vi "TestExec.Config, Dialog, Setup Station Config.vi"(7 "Error if EXE does not exist":bool, 8 "Error if File Doesn't Exist":bool, 9 "Create File if Doesn't Exist":bool, 11 "Path":path=path "C:/MTE/Test Executive/Config") -> (0 "error out":errorcluster, 1 "Station IP Port":i32, 2 "Station Name":string, 3 "Sta Exe Path":path)   [LabVIEW 2018]
uses:
  <vilib>/Utility/config.llb/Read Key (String).vi
  <vilib>/Utility/config.llb/Read Key (I32).vi
  <vilib>/Utility/config.llb/Read Key (Path).vi
  <vilib>/Utility/config.llb/NI_LVConfig.lvlib
  <vilib>/KATE/Files/File Utils.lvlib
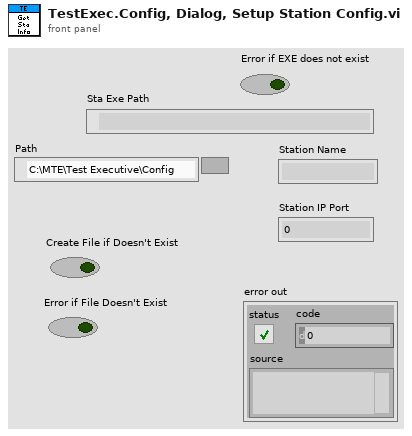
[diagram p1: front panel]
types:
  T1 = typedef "NI_LVConfig.lvlib/Config Data RefNum.ctl" = refnum<k1>
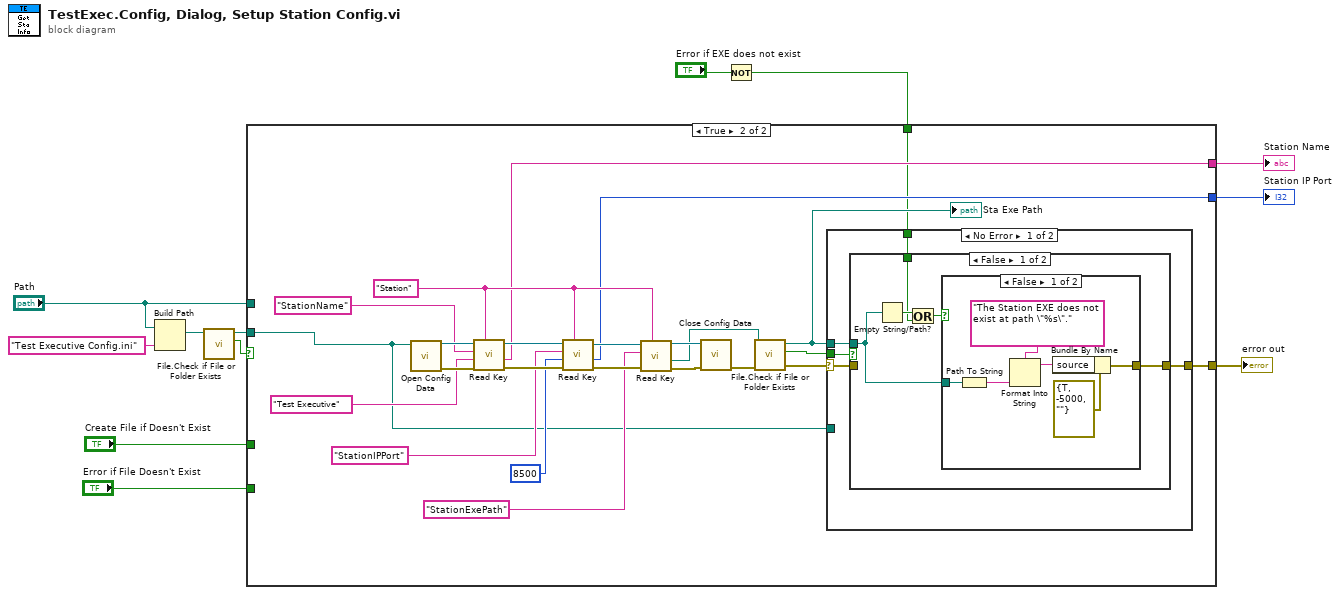
[diagram p0: block diagram]
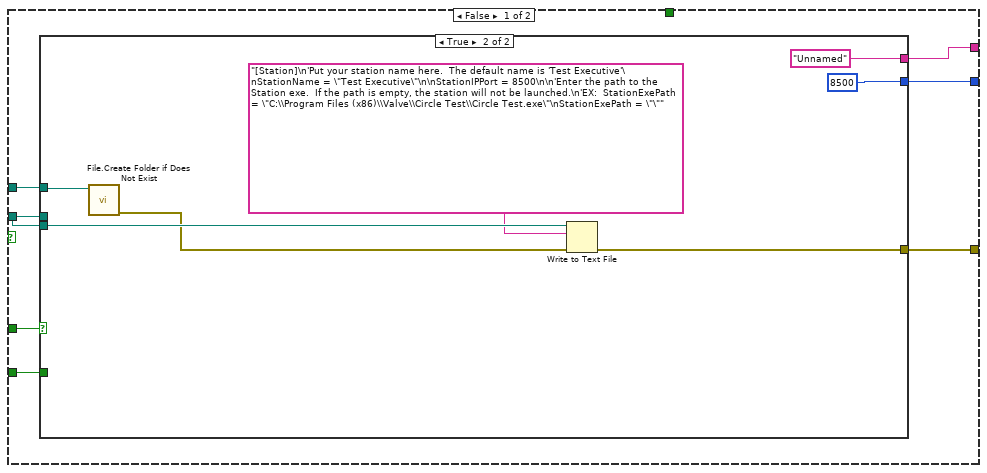
[diagram p2: hidden frame]
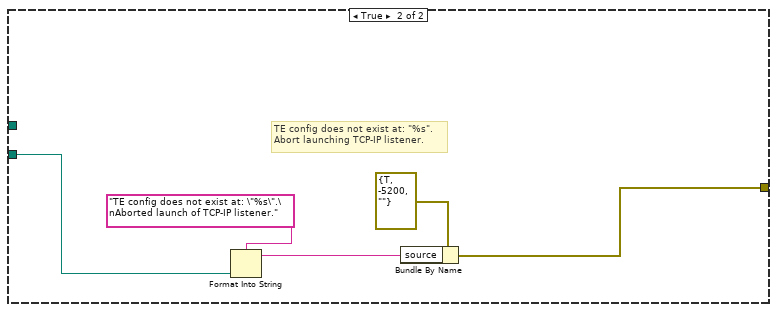
[diagram p4: hidden frame]
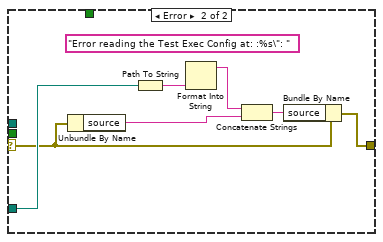
[diagram p7: hidden frame]
diagram:
  n1 = Build Path(base path="Path", name or relative path="Test Executive Config.ini") -> (appended path=w10:path)
  n2 = call <vilib>:"File.Check if File or Folder Exists.vi"("Path"=w10) -> ("Exists"=w8:bool, "Dup Path"=w9:path)  [unwired: 6 in, 3 out]
  n3 = Not(x="Error if EXE does not exist") -> (.not. x?=w1:bool)
  n4 = case shown="True" w8 {
    tunnel: [w19 w56] -> w12
    tunnel: w9 -> [w14 w39]
    tunnel: "Create File if Doesn't Exist" -> [w18 _]
    tunnel: [w16 w38] -> w6
    tunnel: [w17 w37] -> w5
    tunnel: "Error if File Doesn't Exist" -> [w15 _]
    tunnel: "Path" -> [w13 _]
    tunnel: w1 -> [_ w36]
    frame False {
      n5 = case shown="True" w18 {
        tunnel: w14 -> [_ w35]
        tunnel: [w21 w33] -> w19
        tunnel: [_ 8500] -> w17
        tunnel: [_ "Unnamed"] -> w16
        tunnel: w15 -> [w23 _]
        tunnel: w14 -> [w22 _]
        tunnel: w13 -> [w20 w30]
        frame False {
          n6 = case shown="False" w23 {
            tunnel: w22 -> [_ w27]
            tunnel: [_ w24] -> w21
            tunnel: w20 -> [_ _]
            frame False {
            }
            frame True {
              # "TE config does not exist at: \"%s\".\nAbort launching TCP-IP listener."
              n7 = Format Into String(format string="TE config does not exist at: \"%s\".\nAborted launch of TCP-IP listener." ("source"), w27) -> (resulting string=w25:string)  [unwired: 2 in, 1 out]
              n8 = Bundle By Name(cluster=errorcluster {"status"=TRUE, "code"=-5200, "source"=""} ("error constant"), "source"=w25) -> (w24:errorcluster)
            }
          }
        }
        frame True {
          n9 = call <vilib>:"File.Create Folder if Does Not Exist.vi"("Path"=w30) -> ("error out"=w29:errorcluster)  [unwired: 8 in, 2 out]
          n10 = Write to Text File(file (use dialog)=w35, text="[Station]\n'Put your station name here.  The default name is 'Test Executive'\nStationName = \"Test Executive\"\n\nStationIPPort = 8500\n\n'Enter the path to the Station exe.  If the path is empty, the station will not be launched.\n'EX:  StationExePath = \"C:\\Program Files (x86)\\Valve\\Circle Test\\Circle Test.exe\"\nStationExePath = \"\"", error in=w29) -> (error out=w33:errorcluster)  [unwired: 1 in, 2 out]
        }
      }
    }
    frame True {
      w45 = "Station" ("section")
      n11 = call <vilib>:"Open Config Data.vi"("configuration file path"=w39) -> ("error out"=w53:errorcluster, "refnum"=w54:T1)  [unwired: 8 in, 1 out]
      n12 = call-poly <vilib>:"Read Key.vi"("section"=w45, "error in (no error)"=w53, "default value"="Test Executive" ("section"), "key"="StationName" ("section"), "refnum"=w54) -> ("error out"=w52:errorcluster, "value"=w38:string, "refnum out"=w51:T1)  [unwired: 3 in, 1 out]
      n13 = call-poly <vilib>:"Read Key.vi"("section"=w45, "error in (no error)"=w52, "default value"=8500, "key"="StationIPPort", "refnum"=w51) -> ("error out"=w48:errorcluster, "value"=w37:i32, "refnum out"=w49:T1)  [unwired: 3 in, 1 out]
      n14 = call-poly <vilib>:"Read Key.vi"("section"=w45, "error in (no error)"=w48, "key"="StationExePath", "refnum"=w49) -> ("error out"=w47:errorcluster, "value"=w41:path, "refnum out"=w46:T1)  [unwired: 4 in, 1 out]
      n15 = call <vilib>:"Close Config Data.vi"("error in (no error)"=w47, "refnum"=w46) -> ("error out"=w59:errorcluster)  [unwired: 8 in, 1 out]
      n16 = call <vilib>:"File.Check if File or Folder Exists.vi"("error in"=w59, "Path"=w41) -> ("error out"=w58:errorcluster, "Exists"=w57:bool, "Dup Path"=w55:path)  [unwired: 5 in, 2 out]
      "Sta Exe Path" <- w55
      n17 = case shown="No Error" w58 {
        selector: w58 -> [w62 w78]
        tunnel: w57 -> [w64 _]
        tunnel: w55 -> [w63 _]
        tunnel: [w61 w77] -> w56
        tunnel: w39 -> [_ w82]
        tunnel: w36 -> [w60 _]
        frame No Error {
          n18 = case shown="False" w64 {
            tunnel: w63 -> [w68 _]
            tunnel: w62 -> [_ w76]
            tunnel: [w69 w76] -> w61
            tunnel: w60 -> [w65 _]
            frame False {
              n19 = Empty String/Path?(string/path=w68) -> (empty?=w67:bool)
              n20 = Or(x=w67, y=w65) -> (x .or. y?=w66:bool)
              n21 = case shown="False" w66 {
                tunnel: [w71 _] -> w69
                tunnel: w68 -> [w70 _]
                frame False {
                  n22 = Path To String(path=w70) -> (string=w75:string)
                  n23 = Format Into String(format string="The Station EXE does not exist at path \"%s\".", w75) -> (resulting string=w73:string)  [unwired: 2 in, 1 out]
                  n24 = Bundle By Name(cluster=errorcluster {"status"=TRUE, "code"=-5000, "source"=""} ("error constant"), "source"=w73) -> (w71:errorcluster)
                }
                frame True {
                }
              }
            }
            frame True {
            }
          }
        }
        frame Error {
          (unwired) "Error reading the Test Exec Config at: :%s\": "
          n25 = Unbundle By Name(w78) -> ("source"=w80:string)
          n26 = Path To String(path=w82) -> (string=w83:string)
          n27 = Format Into String(w83) -> (resulting string=w81:string)  [unwired: 3 in, 1 out]
          n28 = Concatenate Strings(w81, w80) -> (w79:string)
          n29 = Bundle By Name(cluster=w78, "source"=w79) -> (w77:errorcluster)
        }
      }
    }
  }
  "error out" <- w12
  "Station Name" <- w6
  "Station IP Port" <- w5
